vi "CellDirtyStateChanged Event Callback.vi"(4 "DataGridView in":refnum<class "DataGridView.lvclass">, 5 "Event Data":cluster{"sender":refnum<k24>, "e":refnum<k24>}, 6 "Control Ref":refnum<k24>, 7 "Event Common Data":T1) -> ()   [LabVIEW 2020, in "DataGrid.lvlib" / "DataGridView.lvclass"]
uses:
  DataGridView/DataGridView.lvclass
  System.Windows.Forms
  CellDirtyStateChanged/CellDirtyStateChanged.lvclass
  C:/GEECS/Developers Version/source/Shared/LabVIEWdotNetDataGrid-master/source/Events/Abstract EVENT/Abstract EVENT.lvclass
  CellDirtyStateChanged/CellDirtyStateChanged.lvclass/CellDirtyStateChanged.ctl
  CellDirtyStateChanged/Write cell value.vi
  CellDirtyStateChanged/Write row.vi
  CellDirtyStateChanged/Write column.vi
  CellDirtyStateChanged/Write Dirty.vi
panel:
  out "CommitEdit":bool
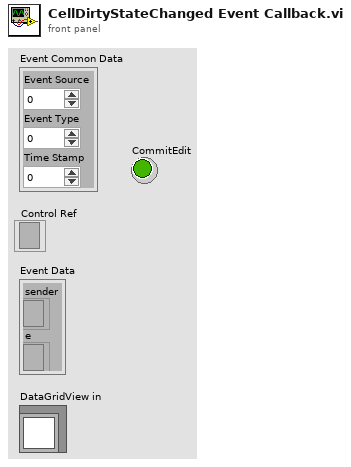
[diagram p1: front panel]
types:
  T1 = cluster{"Event Source":i32, "Event Type":u32, "Time Stamp":u32}
  T2 = cluster{"CellClicked":refnum<user-event>, "CellValue Changed":refnum<user-event>, "KeyDown":refnum<user-event>, "DataError":refnum<user-event>, "UserAddedRow":refnum<user-event>, "UserDeletedRow":refnum<user-event>, "CellDirtyStateChanged":refnum<user-event>}
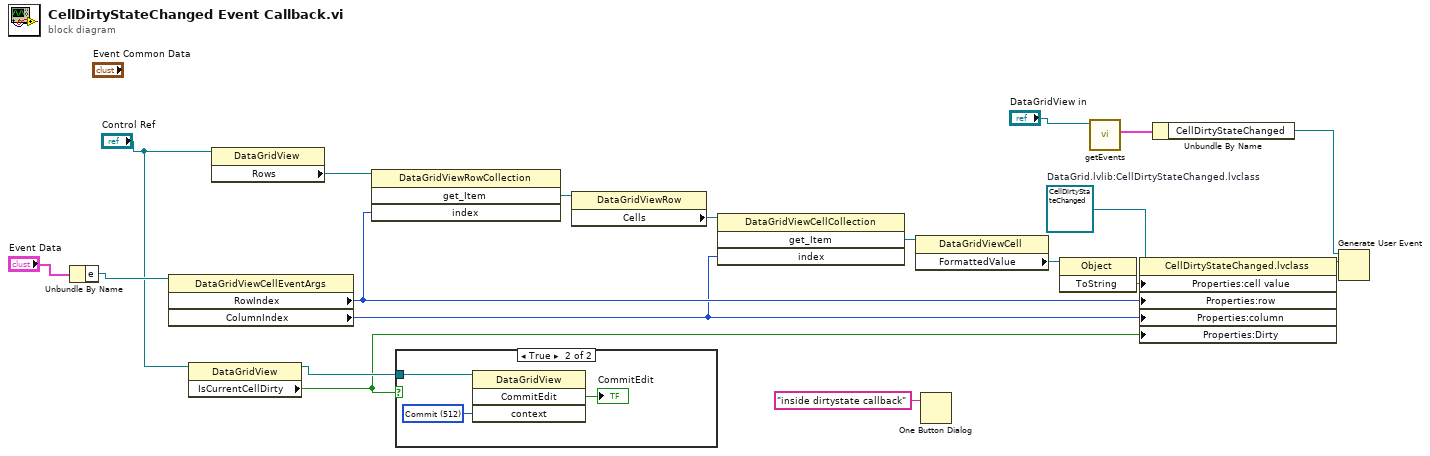
[diagram p0: block diagram]
diagram:
  w8 = refnum<class "CellDirtyStateChanged.lvclass"> refnum  # DataGrid.lvlib:CellDirtyStateChanged.lvclass
  n1 = Unbundle By Name("Event Data") -> ("e"=w5:refnum<k24>)
  n2 = property class="DataGridViewCellEventArgs"(reference=w5) -> ("RowIndex"=w16:i32, "ColumnIndex"=w13:i32)  [unwired: 1 in, 2 out]
  n3 = property class="DataGridView"(reference="Control Ref") -> (reference out=w7:refnum<k24>, "IsCurrentCellDirty"=w2:bool)  [unwired: 1 in, 1 out]
  n4 = property class="DataGridView"(reference="Control Ref") -> ("Rows"=w17:refnum<k24>)  [unwired: 1 in, 2 out]
  n5 = invoke class="DataGridViewRowCollection" method="get_Item"(reference=w17, "index"=w16) -> ("get_Item"=w15:refnum<k24>)  [unwired: 2 in, 3 out]
  n6 = case shown="True" w2 {
    tunnel: w7 -> [_ w22]
    frame False {
    }
    frame True {
      w21 = 512 items=["Formatting"=1, "Display"=2, "PreferredSize"=4, "RowDeletion"=8, "Parsing"=256, "Commit"=512, "InitialValueRestoration"=1024, "LeaveControl"=2048, "CurrentCellChange"=4096, "Scroll"=8192, "ClipboardContent"=16384] ("context")
      n7 = invoke class="DataGridView" method="CommitEdit"(reference=w22, "context"=w21) -> ("CommitEdit"=→"CommitEdit":bool)  [unwired: 2 in, 3 out]
    }
  }
  n8 = property class="DataGridViewRow"(reference=w15) -> ("Cells"=w14:refnum<k24>)  [unwired: 1 in, 2 out]
  n9 = invoke class="DataGridViewCellCollection" method="get_Item"(reference=w14, "index"=w13) -> ("get_Item"=w12:refnum<k24>)  [unwired: 2 in, 3 out]
  n10 = property class="DataGridViewCell"(reference=w12) -> ("FormattedValue"=w11:refnum<k24>)  [unwired: 1 in, 2 out]
  n11 = One Button Dialog(message="inside dirtystate callback") -> ()  [unwired: 1 in, 1 out]
  n12 = invoke class="Object" method="ToString"(reference=w11) -> ("ToString"=w10:string)  [unwired: 2 in, 2 out]
  n13 = call "getEvents.vi"("DataGridView in"="DataGridView in") -> ("userEvents"=w19:T2)  [unwired: 8 in, 2 out]
  n14 = property class="CellDirtyStateChanged.lvclass"(reference=w8, "Properties:cell value"=w10, "Properties:row"=w16, "Properties:column"=w13, "Properties:Dirty"=w2) -> (reference out=w9:refnum<class "CellDirtyStateChanged.lvclass">)  [unwired: 1 in, 1 out]
  n15 = Unbundle By Name(w19) -> ("CellDirtyStateChanged"=w18:refnum<user-event>)
  n16 = Generate User Event(user event=w18, event data cluster=w9) -> ()  [unwired: 2 in, 2 out]
